vi "Pull Remote Branch.vi"(8 "error in":errorcluster, 11 "Peer Review":refnum<class "Peer Review.lvclass">) -> (0 "error out":errorcluster)   [LabVIEW 2020, in "Peer Review.lvclass"]
uses:
  Peer Review.lvclass
  Peer Review.lvclass/Peer Review.ctl
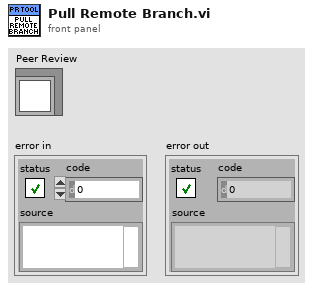
[diagram p1: front panel]
types:
  T1 = enum32{"Commit History", "File List", "Git Log", "Description", "Image"}
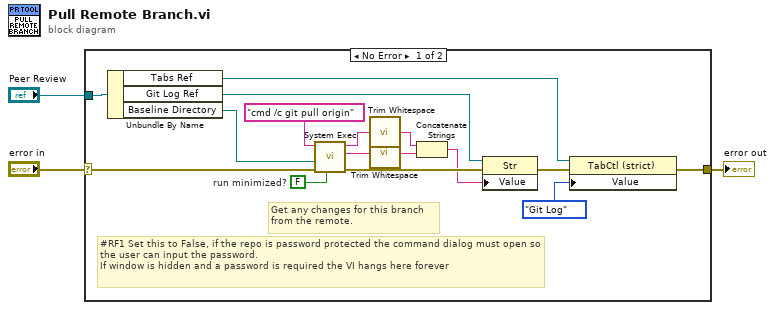
[diagram p0: block diagram]
diagram:
  n1 = case shown="No Error" "error in" {
    selector: "error in" -> [w18 w20]
    tunnel: [w15 w20] -> w2
    tunnel: "Peer Review" -> [w17 _]
    frame No Error {
      w13 = FALSE  # run minimized?
      # "#RF1 Set this to False, if the repo is password protected the command dialog must open so the user can input the password.\nIf window is hidden and a password is required the VI hangs here forever"
      # "Get any changes for this branch\nfrom the remote."
      n2 = Unbundle By Name(w17) -> ("Tabs Ref"=w14:refnum<vi>, "Git Log Ref"=w16:refnum<vi>, "Baseline Directory"=w19:path)
      n3 = call <vilib>:"System Exec.vi"("run minimized? (F)"=w13, "error in (no error)"=w18, "working directory"=w19, "command line"="cmd /c git pull origin" ("String 2")) -> ("error out"=w10:errorcluster, "standard error"=w9:string, "standard output"=w11:string)  [unwired: 4 in, 1 out]
      n4 = call <vilib>:"Trim Whitespace.vi"("string"=w11) -> ("trimmed string"=w7:string)  [unwired: 1 in]
      n5 = call <vilib>:"Trim Whitespace.vi"("string"=w9) -> ("trimmed string"=w8:string)  [unwired: 1 in]
      n6 = Concatenate Strings(w7, w8) -> (w6:string)
      n7 = property class="Str"(reference=w16, error in=w10, "Value"=w6) -> (error out=w5:errorcluster)  [unwired: 1 out]
      n8 = property on="Property Node" class="TabCtl (strict)"(reference=w14, error in=w5, "Value"=T1."Git Log") -> (error out=w15:errorcluster)  [unwired: 1 out]
    }
    frame Error {
    }
  }
  "error out" <- w2
